vi "Acroname_Port_Disable.vi"(8 "error in (no error)":errorcluster, 11 "Port Number":i32) -> (0 "error out":errorcluster)   [LabVIEW 2025]
uses:
  1b1786e0-183b-4c19-b690-1d9e1fdb2131.vi
  BrainStem2_LabVIEW_Library.lvlib
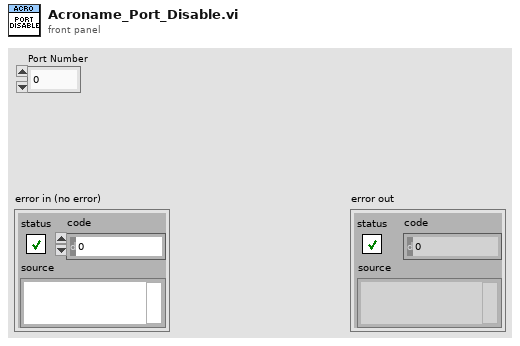
[diagram p1: front panel]
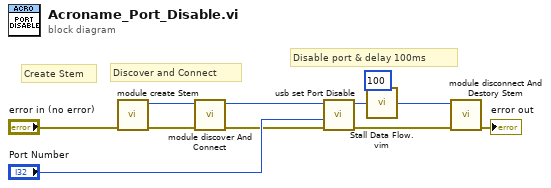
[diagram p0: block diagram]
diagram:
  # "Disable port & delay 100ms"
  # "Discover and Connect"
  # "Create Stem"
  n1 = call "module create Stem.vi"("error in (no error)"="error in (no error)") -> ("error out"=w7:errorcluster, "id out"=w11:u32)  [unwired: 8 in, 1 out]
  n2 = call "module discover And Connect.vi"("error in (no error)"=w7, "id"=w11) -> ("error out"=w6:errorcluster, "id out"=w10:u32)  [unwired: 7 in, 1 out]
  n3 = call "usb set Port Disable.vi"("error in (no error)"=w6, "channel"="Port Number", "id"=w10) -> ("error out"=w4:errorcluster, "id out"=w2:u32)  [unwired: 6 in, 1 out]
  n4 = call "Stall Data Flow.vim"("value in"=w2, "milliseconds to wait"=100) -> ("value out"=w9:u32)  [unwired: 1 out]
  n5 = call "module disconnect And Destory Stem.vi"("error in (no error)"=w4, "id"=w9) -> ("error out"=→"error out":errorcluster)  [unwired: 7 in, 2 out]
